vi "表格适应.vi"(9 "Red-F":bool, 10 "new":string[](array[string])=["11", "22", "33", "44", "55", "66"], 11 "表格in":refnum<vi>) -> ()   [LabVIEW 2015]
uses:
  <vilib>/Utility/miscctls.llb/LVRowAndColumnTypeDef.ctl
  <vilib>/Utility/miscctls.llb/LVRowAndColumnUnsignedTypeDef.ctl
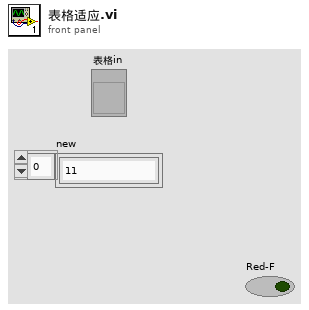
[diagram p1: front panel]
types:
  T1 = typedef "LVRowAndColumnTypeDef.ctl" = cluster{"Row":i32, "Column":i32}
  T2 = typedef "LVRowAndColumnUnsignedTypeDef.ctl" = cluster{"Row":u32, "Column":u32}
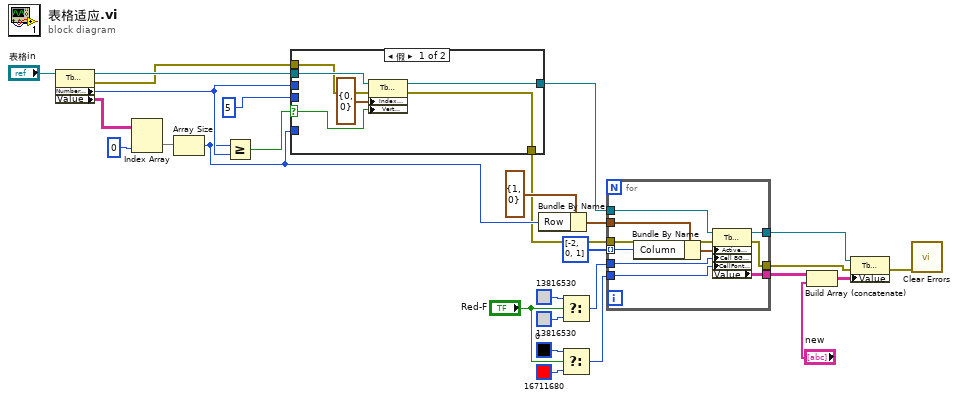
[diagram p0: block diagram]
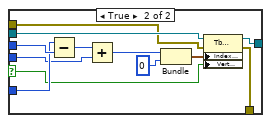
[diagram p2: hidden frame]
diagram:
  n1 = property class="Tbl (严格)"(reference="表格in") -> (reference out=w11:refnum<vi>, error out=w4:errorcluster, "Number of Rows"=w7:u32, "Value"=w14:string[][])  [unwired: 1 in]
  n2 = Index Array(array=w14, index (col)=0 ("禁用的索引 (列)")) -> (element=w12:string[])  [unwired: 1 in]
  n3 = Array Size(array=w12) -> (size(s)=w6:i32)
  n4 = Greater Or Equal?(x=w6, y=w7) -> (x >= y?=w10:bool)
  n5 = case shown="假" w10 {
    selector: w10 -> [w32 w38]
    tunnel: w11 -> [w34 w46]
    tunnel: 5 ("RowMax") -> [_ w40]
    tunnel: w7 -> [_ w43]
    tunnel: w6 -> [_ w42]
    tunnel: [w31 w37] -> w8
    tunnel: w4 -> [w30 w36]
    tunnel: [w29 w35] -> w3
    frame False {
      n6 = property class="Tbl (严格)"(reference=w34, error in=w30, "Index Values"=T2 {"Row"=0, "Column"=0} ("索引值"), "Vert Scrollbar"=w32) -> (reference out=w31:refnum<vi>, error out=w29:errorcluster)
    }
    frame True {
      n7 = Subtract(x=w42, y=w43) -> (x-y=w41:u32)
      n8 = Add(x=w41, y=w40) -> (x+y=w39:u32)
      n9 = Bundle(w39, "禁用的索引 (列)"=0) -> (w45:cluster{u32, "禁用的索引 (列)":i32})  [unwired: 1 in]
      n10 = property class="Tbl (严格)"(reference=w46, error in=w36, "Index Values"=w45, "Vert Scrollbar"=w38) -> (reference out=w37:refnum<vi>, error out=w35:errorcluster)
    }
  }
  n11 = Bundle By Name(cluster=T1 {"Row"=1, "Column"=0} ("活动单元格:活动单元格"), "Row"=w6) -> (w24:T1)
  n12 = Select(t=u32 13816530, s="Red-F", f=u32 13816530) -> (s? t:f=w23:u32)
  n13 = Select(t=u32 0, s="Red-F", f=u32 16711680) -> (s? t:f=w19:u32)
  n14 = for {
    tunnel: w8 -> [w56]
    tunnel: i32[] [-2, 0, 1] -> [w53] mode=indexing
    tunnel: w24 -> [w54]
    tunnel: w23 -> [w52]
    tunnel: w19 -> [w51]
    tunnel: [w50] -> w18
    tunnel: [w49] -> w16
    tunnel: w3 -> [w48]
    tunnel: [w47] -> w2
    n15 = Bundle By Name(cluster=w54, "Column"=w53) -> (w55:T1)
    n16 = property class="Tbl (严格)"(reference=w56, error in=w48, "Active Cell"=w55, "Cell BG Color"=w52, "CellFontColor"=w51) -> (reference out=w50:refnum<vi>, error out=w47:errorcluster, "Value"=w49:string[][])
  }
  n17 = Build Array (concatenate)(w16, "new") -> (w17:string[][])
  n18 = property class="Tbl (严格)"(reference=w18, error in=w2, "Value"=w17) -> (error out=w1:errorcluster)  [unwired: 1 out]
  n19 = call <vilib>:"Clear Errors.vi"("error in (no error)"=w1) -> ()  [unwired: 5 in, 2 out]
